vi "DumbDash Save Values.vi"(9 "Message Box":refnum<vi>, 10 "Robot":T1, 11 "Controls In":T2[](array[typedef])) -> ()   [LabVIEW 2017]
uses:
  DumbDash Control.ctl
  DumbDash Control Type.ctl
  Common Code/Robot Name.ctl
  <vilib>/Utility/sysdir.llb/System Directory Type.ctl
  <vilib>/Utility/config.llb/Write Key (Double).vi
  <vilib>/Utility/config.llb/Write Key (Boolean).vi
  <vilib>/Utility/config.llb/Write Key (String).vi
  <vilib>/Utility/config.llb/NI_LVConfig.lvlib
panel:
  out "file created?":bool
  out "file path":path
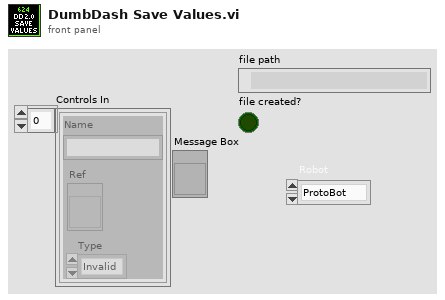
[diagram p1: front panel]
types:
  T1 = typedef "Robot Name.ctl" = enum16{"ProtoBot", "Main Robot", "Practice Robot"}
  T2 = typedef "DumbDash Control.ctl" = cluster{"Name":string, "Ref":refnum<vi>, "Type":T3}
  T3 = typedef "DumbDash Control Type.ctl" = enum16{"Invalid", "Number", "Boolean", "String"}
  T4 = typedef "System Directory Type.ctl" = i32
  T5 = typedef "NI_LVConfig.lvlib/Config Data RefNum.ctl" = refnum<k1>
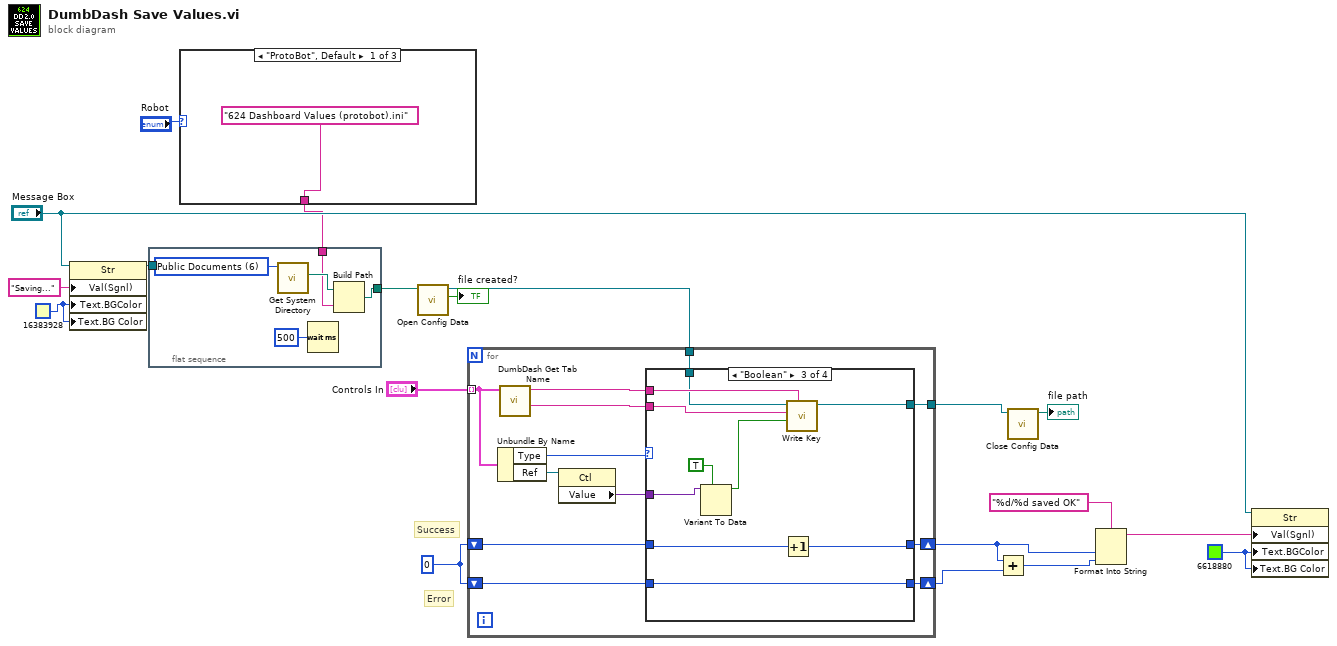
[diagram p0: block diagram]
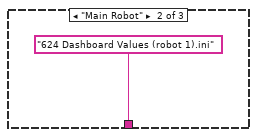
[diagram p2: hidden frame]
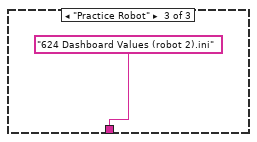
[diagram p3: hidden frame]
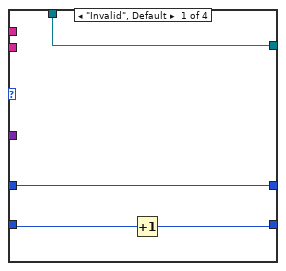
[diagram p4: hidden frame]
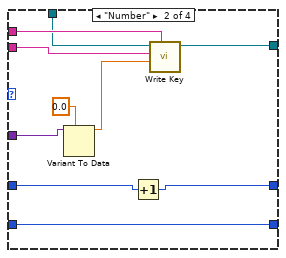
[diagram p5: hidden frame]
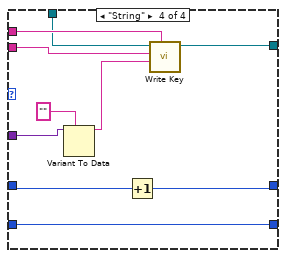
[diagram p6: hidden frame]
diagram:
  w4 = u32 16383928
  w7 = u32 6618880
  w13 = 0
  # "Error"
  # "Success"
  n1 = property class="Str"(reference="Message Box", "Val(Sgnl)"="Saving..." ("Text.Text"), "Text.BGColor"=w4, "Text.BG Color"=w4) -> (reference out=w3:refnum<vi>)  [unwired: 1 in, 1 out]
  n2 = flat-sequence {
    tunnel: [w22] -> w14
    tunnel: w3 -> [_]
    tunnel: w1 -> [w20]
    frame #0 {
      w24 = T4 6 items=["User Home"=0, "User Desktop"=1, "User Documents"=2, "User Application Data"=3, "User Preferences"=4, "User Temporary"=5, "Public Documents"=6, "Public Application Data"=7, "Public Preferences"=8, "Public Cache"=13, "System Core Libraries"=9, "System Installed Libraries"=10, "Application Files"=11, "Boot Volume Root"=12] ("system directory type")
      n3 = call <vilib>:"Get System Directory.vi"("system directory type"=w24) -> ("system directory"=w23:path)  [unwired: 10 in]
      n4 = Wait (ms)(milliseconds to wait=u32 500) -> ()  [unwired: 1 out]
      n5 = Build Path(base path=w23, name or relative path=w20) -> (appended path=w22:path)
    }
  }
  n6 = case shown="\"ProtoBot\", Default" "Robot" {
    tunnel: ["624 Dashboard Values (protobot).ini" ("name or relative path") "624 Dashboard Values (robot 1).ini" ("name or relative path") "624 Dashboard Values (robot 2).ini" ("name or relative path")] -> w1
    frame "ProtoBot", Default {
    }
    frame "Main Robot" {
    }
    frame "Practice Robot" {
    }
  }
  n7 = call <vilib>:"Open Config Data.vi"("configuration file path"=w14) -> ("file created?"=→"file created?":bool, "refnum"=w18:T5)  [unwired: 8 in, 1 out]
  n8 = for {
    tunnel: "Controls In" -> [w35] mode=indexing
    tunnel: w18 -> [w38]
    tunnel: [w32] -> w17
    shift-right: [w28] -> w11
    shift-left: w13 -> [w29]
    shift-right: [w30] -> w10
    shift-left: w13 -> [w31]
    n9 = Unbundle By Name(w35) -> ("Type"=w36:T3, "Ref"=w34:refnum<vi>)
    n10 = call "DumbDash Get Tab Name.vi"("Cluster"=w35) -> ("Rest of Name"=w37:string, "Tab Name"=w39:string)  [unwired: 9 in]
    n11 = property class="Ctl"(reference=w34) -> ("Value"=w33:variant)  [unwired: 1 in, 2 out]
    n12 = case shown="\"Boolean\"" w36 {
      tunnel: w39 -> [_ w53 w63 w73]
      tunnel: w38 -> [w43 w52 w62 w72]
      tunnel: w37 -> [_ w51 w61 w71]
      tunnel: w33 -> [_ w50 w60 w70]
      tunnel: [w43 w47 w57 w67] -> w32
      tunnel: w31 -> [w40 w45 w56 w66]
      tunnel: [w40 w44 w55 w65] -> w30
      tunnel: w29 -> [w42 w46 w54 w64]
      tunnel: [w41 w46 w54 w64] -> w28
      frame "Invalid", Default {
        n13 = Increment(x=w42) -> (x+1=w41:i32)
      }
      frame "Number" {
        n14 = Variant To Data(type=0.0, Variant=w50) -> (data=w48:dbl)  [unwired: 1 in, 1 out]
        n15 = Increment(x=w45) -> (x+1=w44:i32)
        n16 = call-poly <vilib>:"Write Key.vi"("section"=w53, "value"=w48, "key"=w51, "refnum"=w52) -> ("refnum out"=w47:T5)  [unwired: 5 in, 2 out]
      }
      frame "Boolean" {
        n17 = Variant To Data(type=TRUE, Variant=w60) -> (data=w59:bool)  [unwired: 1 in, 1 out]
        n18 = Increment(x=w56) -> (x+1=w55:i32)
        n19 = call-poly <vilib>:"Write Key.vi"("section"=w63, "value"=w59, "key"=w61, "refnum"=w62) -> ("refnum out"=w57:T5)  [unwired: 5 in, 2 out]
      }
      frame "String" {
        n20 = Variant To Data(type="", Variant=w70) -> (data=w69:string)  [unwired: 1 in, 1 out]
        n21 = Increment(x=w66) -> (x+1=w65:i32)
        n22 = call-poly <vilib>:"Write Key.vi"("section"=w73, "value"=w69, "key"=w71, "refnum"=w72) -> ("refnum out"=w67:T5)  [unwired: 5 in, 2 out]
      }
    }
  }
  n23 = Add(x=w10, y=w11) -> (x+y=w9:i32)
  n24 = call <vilib>:"Close Config Data.vi"("refnum"=w17) -> ("file path"=→"file path":path)  [unwired: 9 in, 1 out]
  n25 = Format Into String(format string="%d/%d saved OK", w10, w9) -> (resulting string=w8:string)  [unwired: 2 in, 1 out]
  n26 = property class="Str"(reference="Message Box", "Val(Sgnl)"=w8, "Text.BGColor"=w7, "Text.BG Color"=w7) -> ()  [unwired: 1 in, 2 out]
